vi "DMM_Keysight_34980A_SoftFP.vi"(0 "reference in":refnum<class "DMM_Keysight_34980A.lvclass">, 2 "Floating":bool, 5 "error in (no error)":errorcluster) -> (14 "reference out":refnum<class "DMM_Keysight_34980A.lvclass">, 19 "error out":errorcluster)   [LabVIEW 2022 SP3, in "DMM_Keysight_34980A.lvlib" / "DMM_Keysight_34980A.lvclass"]
uses:
  DMM_Keysight_34980A.lvclass
  Res.ctl
  Mode.ctl
  <vilib>/Analysis/baseanly.llb/Mean (DBL).vi
  Components/ViPER.lvlibp/ViPER.lvclass
  <vilib>/Utility/Data Type/NI_Data Type.lvlib
  C:/Projects/Medulla/ViPER/Examples/Flux_Capacitor_Tester/Components/ViPER.lvlibp/ViPER.lvclass
  <vilib>/Analysis/NI_AALBase.lvlib
panel:
  out "result":dbl
  in  "BW or low F":string(combo) caption="Combo Box"
  in  "Aperature":string(combo) caption="Combo Box"
  in  "Range":string(combo) caption="Combo Box"
  in  "Mode":string(combo) caption="Combo Box"
  in  "Resolution":string(combo) caption="Combo Box"
  in  "Timeout (s)":dbl=10.0 caption="Numeric" min=10.0 max=360.0 step=1.0
  in  "dt (s)":dbl=0.001 caption="Numeric" min=0.001 max=1.0 step=0.001 format="%_1g"
  in  "Samples":u32=1 caption="Numeric" min=1 max=1500 step=1
  in  "Measure":bool
  out "XY Graph":cluster{"Time":dbl[], "Measurement":dbl[]}(graph)
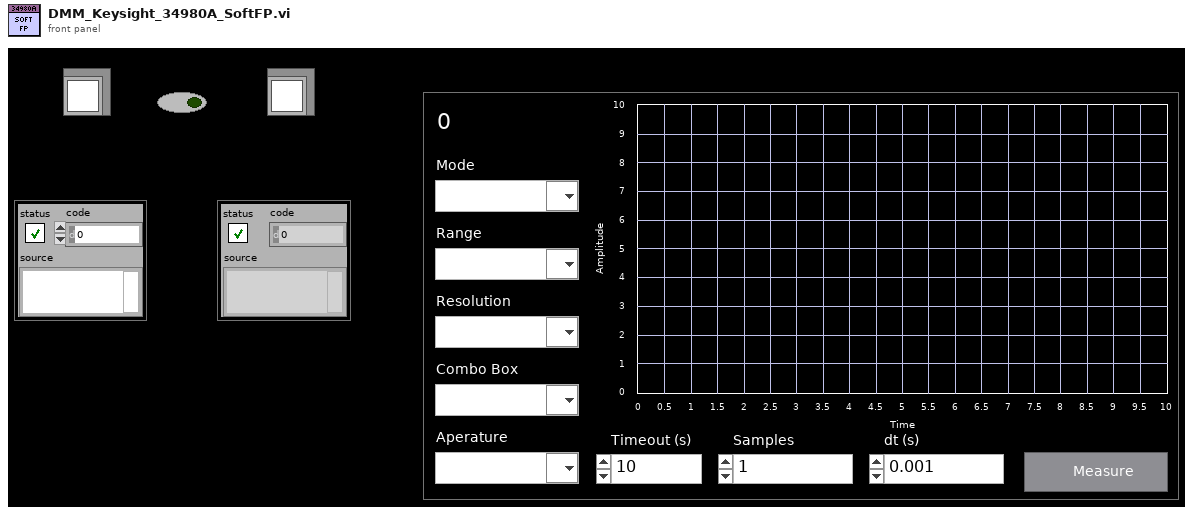
[diagram p1: front panel]
types:
  T1 = enum32{"Invalid", "Standard", "Closed", "Hidden", "Minimized", "Maximized"}
  T2 = enum16{"100 mV", "1 V", "10 V", "100 V", "300 V", "Auto", "Minimum", "Maximum"}
  T3 = enum16{"4 1/2", "5 1/2", "6 1/2", "Least", "Highest", "Default"}
  T4 = enum16{"3 Hz", "20 Hz", "200 Hz", "Minimum", "Maximum"}
  T5 = enum16{"100 mV", "1 V", "10 V", "100 V", "300 V", "Auto", "Minimum", "Maximum", "Default"}
  T6 = enum16{"100 Ohm", "1 kOhm", "10 kOhm", "100 kOhm", "1 MOhm", "10 MOhm", "100 MOhm", "Auto", "Minimum", "Maximum"}
  T7 = enum16{"10 ms", "100 ms", "1 sec", "Minimum", "Maximum"}
  T8 = enum16{"10 mA", "100 mA", "1 A", "Auto", "Minimum", "Maximum"}
  T9 = enum16{"3 Hz", "20 Hz", "200 Hz", "Minimum", "Maximum", "Default"}
  T10 = typedef "DMM_Keysight_34980A.lvlib/DMM_Keysight_34980A.lvclass/Mode.ctl" = enum16{"DCV", "ACV", "2W Ohms", "4W Ohms", "Frequency", "DCA", "ACA"}
  T11 = typedef "DMM_Keysight_34980A.lvlib/DMM_Keysight_34980A.lvclass/Res.ctl" = enum16{"4 1/2", "5 1/2", "6 1/2", "Least", "Highest", "Default"}
  T12 = typedef "DMM_Keysight_34980A.lvlib/DMM_Keysight_34980A.lvclass/ObjectAttributes.ctl" = cluster{"Config":T13, "VISA ref":refnum<visa-resource-name>, "Meas":dbl, "Range DCV":enum16{"100 mV", "1 V", "10 V", "100 V", "300 V", "Auto", "Minimum", "Maximum"}, "Range ACV":enum16{"100 mV", "1 V", "10 V", "100 V", "300 V", "Auto", "Minimum", "Maximum", "Default"}, "Range Ohms":enum16{"100 Ohm", "1 kOhm", "10 kOhm", "100 kOhm", "1 MOhm", "10 MOhm", "100 MOhm", "Auto", "Minimum", "Maximum"}, "Range VFreq":enum16{"100 mV", "1 V", "10 V", "100 V", "300 V", "Auto", "Minimum", "Maximum"}, " Range ACA":enum16{"10 mA", "100 mA", "1 A", "Auto", "Minimum", "Maximum"}, " Range DCA":enum16{"10 mA", "100 mA", "1 A", "Auto", "Minimum", "Maximum"}, "Mode":T10, "Resolution":enum16{"4 1/2", "5 1/2", "6 1/2", "Least", "Highest", "Default"}, "Bandwidth":enum16{"3 Hz", "20 Hz", "200 Hz", "Minimum", "Maximum"}, "Low Frequency":enum16{"3 Hz", "20 Hz", "200 Hz", "Minimum", "Maximum"}, "Aperture":enum16{"10 ms", "100 ms", "1 sec", "Minimum", "Maximum"}, "Measurement":dbl[], "Time":dbl[], "Samples":u32, "dt":dbl, "Timeout":dbl}
  T13 = typedef "DMM_Keysight_34980A.lvlib/DMM_Keysight_34980A.lvclass/Config.ctl" = cluster{"VISA":refnum<visa-resource-name>}
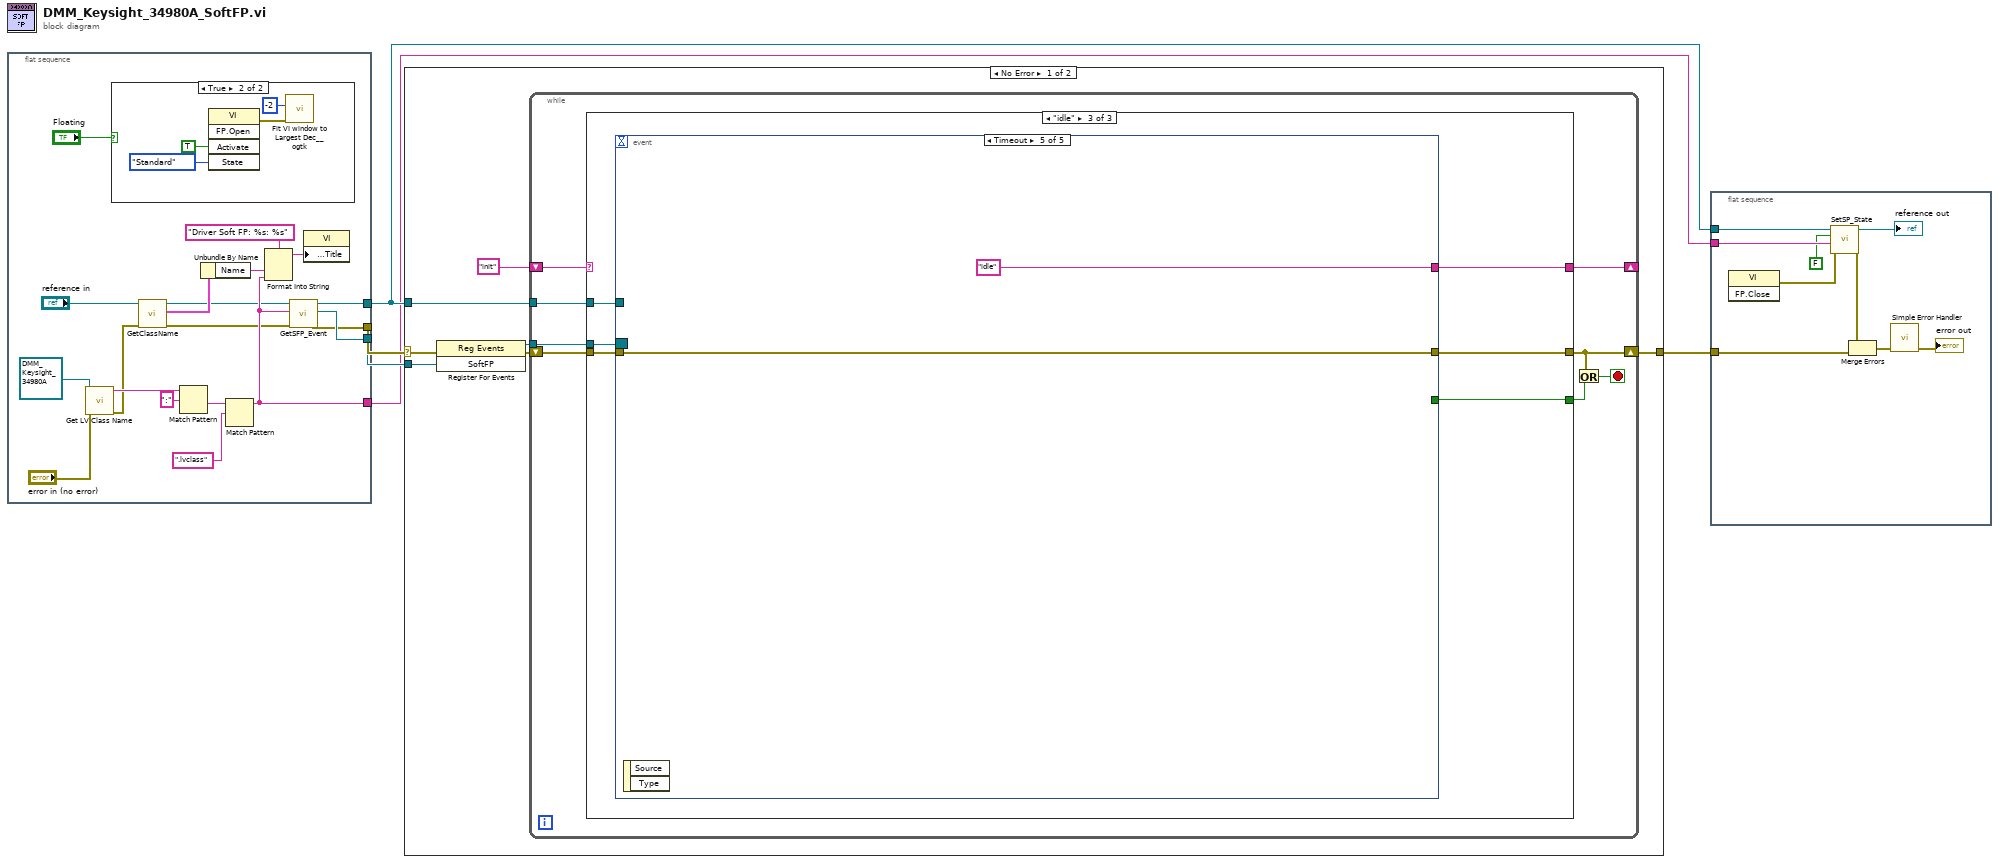
[diagram p0: block diagram]
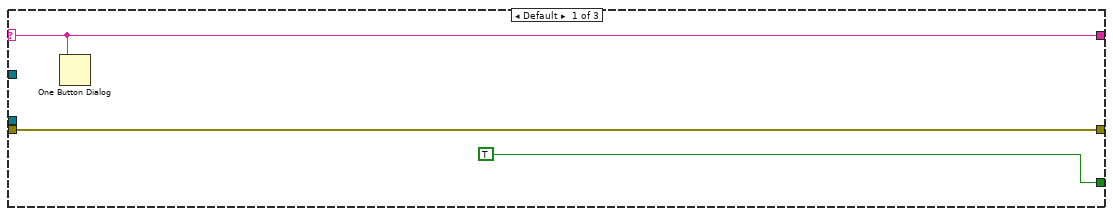
[diagram p3: hidden frame]
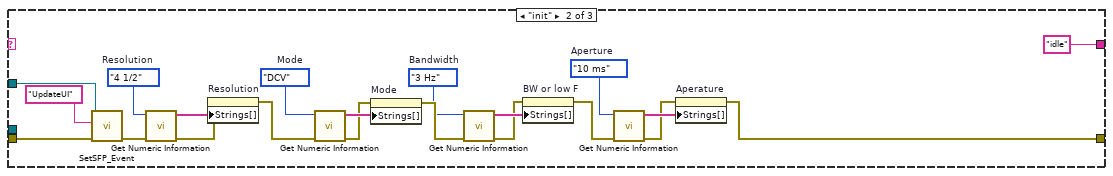
[diagram p4: hidden frame]
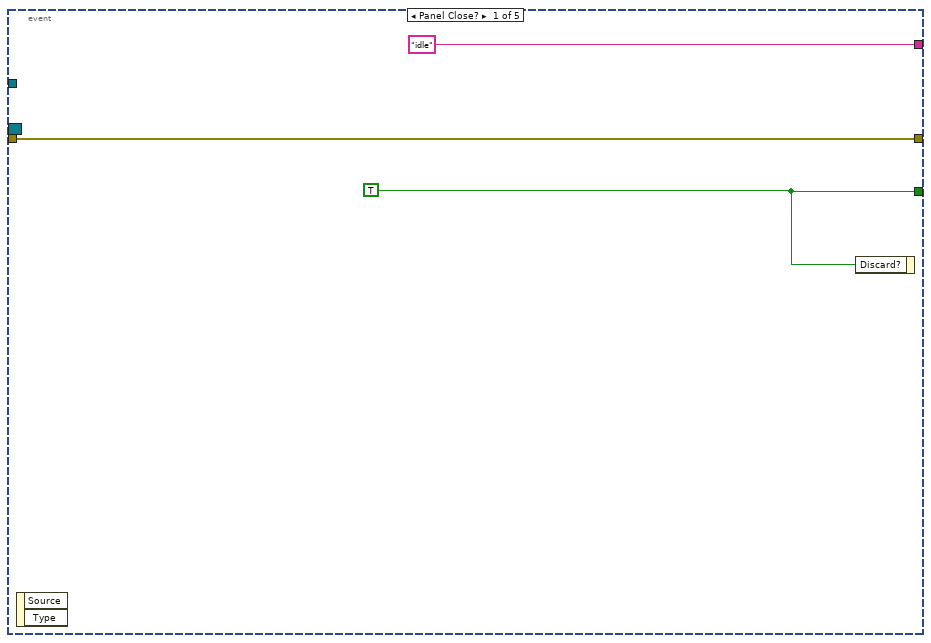
[diagram p5: hidden frame]
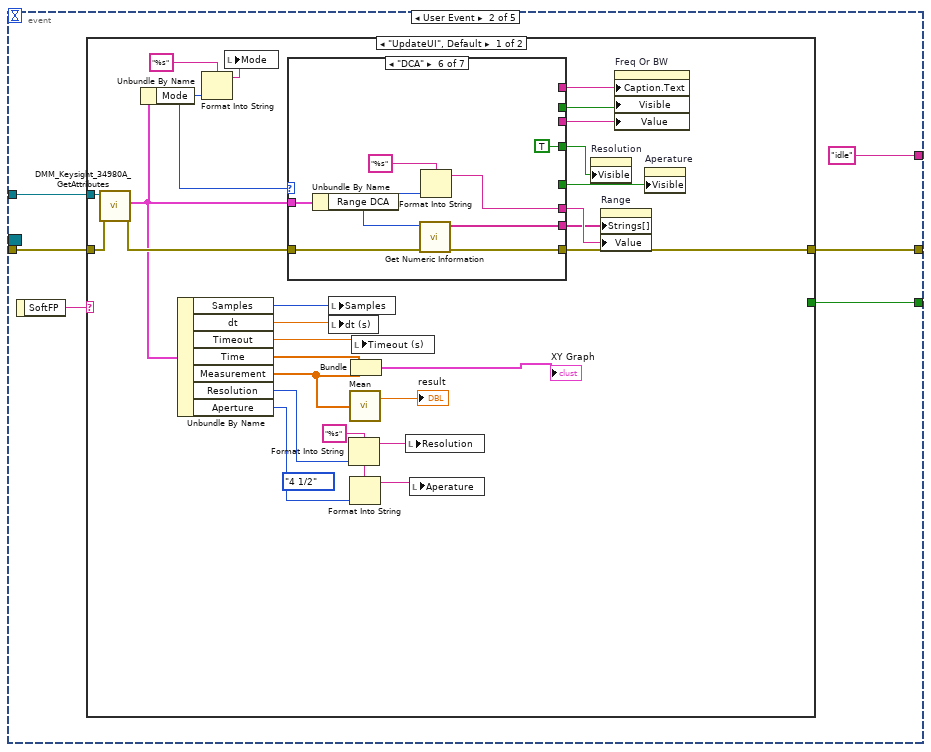
[diagram p6: hidden frame]
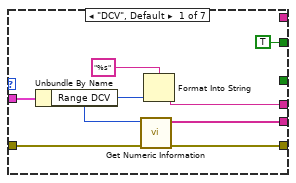
[diagram p7: hidden frame]
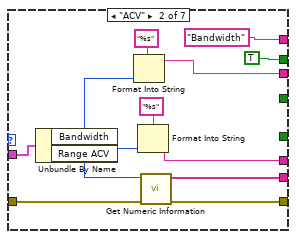
[diagram p8: hidden frame]
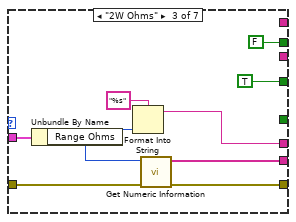
[diagram p9: hidden frame]
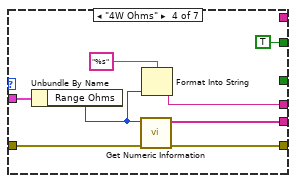
[diagram p10: hidden frame]
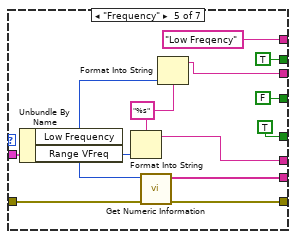
[diagram p11: hidden frame]
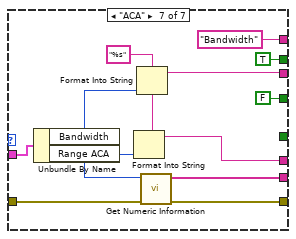
[diagram p12: hidden frame]
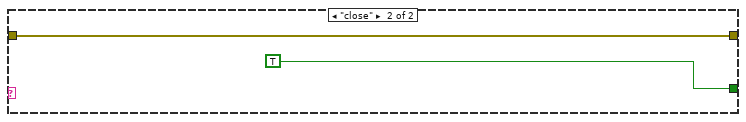
[diagram p13: hidden frame]
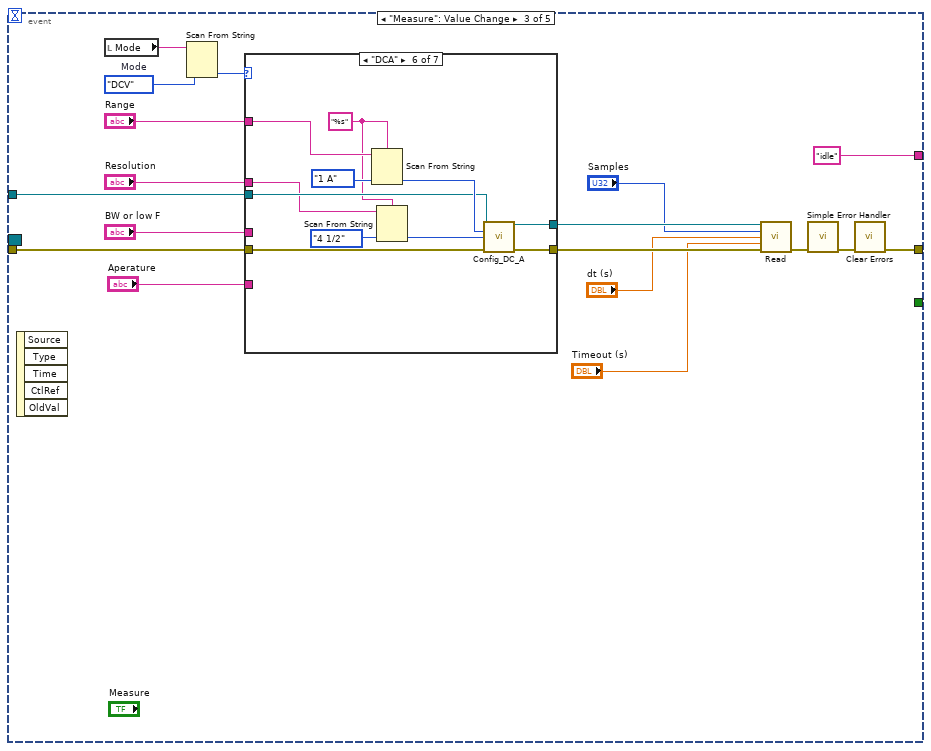
[diagram p14: hidden frame]
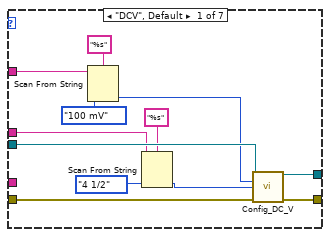
[diagram p15: hidden frame]
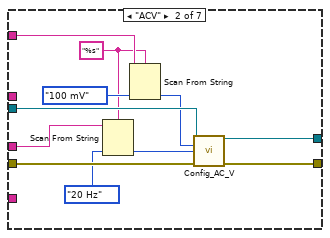
[diagram p16: hidden frame]
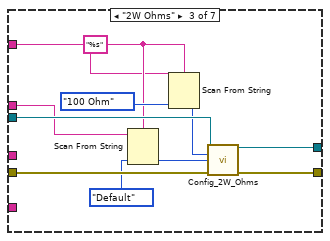
[diagram p17: hidden frame]
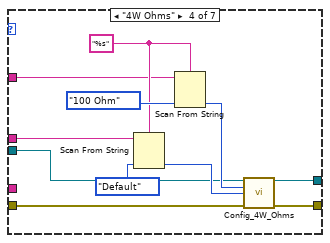
[diagram p18: hidden frame]
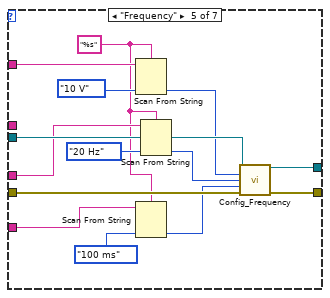
[diagram p19: hidden frame]
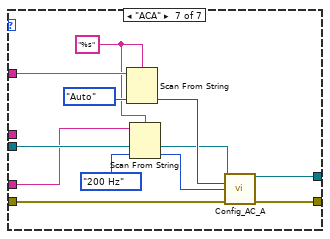
[diagram p20: hidden frame]
diagram:
  n1 = flat-sequence {
    tunnel: [w21] -> w5
    tunnel: [w20] -> w2
    tunnel: [w24] -> w3
    tunnel: [w12] -> w1
    frame #0 {
      n2 = call <vilib>:"Get LV Class Name.vi"("error in (no error)"="error in (no error)", "object"=refnum<class "DMM_Keysight_34980A.lvclass"> refnum ("reference")) -> ("error out"=w11:errorcluster, "class name"=w17:string)  [unwired: 8 in]
      n3 = case shown="True" "Floating" {
        frame False {
        }
        frame True {
          n4 = invoke class="VI" method="FP.Open"("Activate"=TRUE ("Activate?"), "State"=T1."Standard") -> (error out=w25:errorcluster)  [unwired: 3 in, 4 out]
          n5 = call <userlib>:"Fit VI window to Largest Dec__ogtk.vi"("error in (no error)"=w25, "border spacing (2 px)"=-2) -> ()  [unwired: 4 in, 2 out]
        }
      }
      n6 = call "GetClassName.vi"("error in (no error)"=w11, "reference in"="reference in") -> ("error out"=w10:errorcluster, "Details"=w9:cluster{"Name":string, "Class":string}, "reference out"=w7:refnum<class "DMM_Keysight_34980A.lvclass">)  [unwired: 7 in]
      n7 = Match Pattern(string=w17, regular expression=":") -> (after substring=w15:string)  [unwired: 1 in, 3 out]
      n8 = Unbundle By Name(w9) -> ("Name"=w19:string)
      n9 = Match Pattern(string=w15, regular expression=".lvclass") -> (before substring=w12:string)  [unwired: 1 in, 3 out]
      n10 = Format Into String(format string="Driver Soft FP: %s: %s", w19, w12) -> (resulting string=w23:string)  [unwired: 2 in, 1 out]
      n11 = call-dynamic "GetSFP_Event.vi"("error in (no error)"=w10, "Ancestor"=w12, "reference in"=w7) -> ("error out"=w21:errorcluster, "SoftFP"=w24:refnum<user-event>, "reference out"=w20:refnum<class "DMM_Keysight_34980A.lvclass">)  [unwired: 6 in]
      n12 = property class="VI"("Front Panel.Title"=w23) -> ()  [unwired: 2 in, 2 out]
    }
  }
  n13 = case shown="No Error" w5 {
    selector: w5 -> [w33 w301]
    tunnel: [w29 w301] -> w4
    tunnel: w2 -> [w30 _]
    tunnel: w3 -> [w35 _]
    frame No Error {
      n14 = register-events(error in=w33, w35) -> (reference out=w34:refnum<event-registration>, error out=w32:errorcluster)  [unwired: 1 in]
      n15 = while {
        shift-right: [w40] -> w29
        shift-left: w32 -> [w43]
        tunnel: w34 -> [w42]
        tunnel: w30 -> [w41]
        shift-right: [w36] -> _
        shift-left: "init" -> [w37]
        stop <- w39 stop-if-true
        n16 = case shown="\"idle\"" w37 {
          selector: w37 -> [w44 _ _]
          tunnel: w43 -> [w45 w66 w73]
          tunnel: w42 -> [_ _ w72]
          tunnel: w41 -> [_ w65 w71]
          tunnel: [w45 w47 w70] -> w40
          tunnel: [TRUE ("Discard?") _ w69] -> w38
          tunnel: [w44 "idle" w68] -> w36
          frame Default {
            n17 = One Button Dialog(message=w44) -> ()  [unwired: 1 in, 1 out]
          }
          frame "init" {
            w50 = T7."10 ms"  # Aperture
            w54 = T4."3 Hz"  # Bandwidth
            w58 = Mode."DCV"  # Mode
            w62 = Res."4 1/2"  # Resolution
            n18 = call-dynamic "SetSFP_Event.vi"("error in (no error)"=w66, "msg"="UpdateUI", "reference in"=w65) -> ("error out"=w63:errorcluster)  [unwired: 7 in, 1 out]
            n19 = call <vilib>:"Get Numeric Information.vi"("error in (no error)"=w63, "variant"=w62) -> ("error out"=w60:errorcluster, "enum names"=w61:string[])  [unwired: 6 in, 2 out]
            n20 = property on="Resolution" class="CmbBox"(error in=w60, "Strings[]"=w61) -> (error out=w59:errorcluster)  [unwired: 1 in, 1 out]
            n21 = call <vilib>:"Get Numeric Information.vi"("error in (no error)"=w59, "variant"=w58) -> ("error out"=w56:errorcluster, "enum names"=w57:string[])  [unwired: 6 in, 2 out]
            n22 = property on="Mode" class="CmbBox"(error in=w56, "Strings[]"=w57) -> (error out=w55:errorcluster)  [unwired: 1 in, 1 out]
            n23 = call <vilib>:"Get Numeric Information.vi"("error in (no error)"=w55, "variant"=w54) -> ("error out"=w52:errorcluster, "enum names"=w53:string[])  [unwired: 6 in, 2 out]
            n24 = property on="BW or low F" class="CmbBox"(error in=w52, "Strings[]"=w53) -> (error out=w51:errorcluster)  [unwired: 1 in, 1 out]
            n25 = call <vilib>:"Get Numeric Information.vi"("error in (no error)"=w51, "variant"=w50) -> ("error out"=w48:errorcluster, "enum names"=w49:string[])  [unwired: 6 in, 2 out]
            n26 = property on="Aperature" class="CmbBox"(error in=w48, "Strings[]"=w49) -> (error out=w47:errorcluster)  [unwired: 1 in, 1 out]
          }
          frame "idle" {
            n27 = event shown="[4] Timeout" {
              selector: w72 -> [_ _ _ _ _]
              dyn-events: _ -> [_ _ _ _ _]
              timeout: _ -> [_ _ _ _ _]
              tunnel: w73 -> [w76 w82 w199 w289 w300]
              tunnel: [w76 w80 w184 w291 w300] -> w70
              tunnel: [w75 w79 _ _ _] -> w69
              tunnel: w71 -> [_ w77 w198 w288 _]
              tunnel: ["idle" "idle" "idle" "idle" "idle"] -> w68
              event Panel Close? {
                w75 = TRUE ("Discard?")
                n28 = event-data() -> ()  [unwired: 1 in, 2 out]
                n29 = event-data("Discard?"=w75) -> ()  [unwired: 1 in, 1 out]
              }
              event User Event {
                n30 = event-data() -> ("SoftFP"=w81:string)  [unwired: 1 in]
                n31 = case shown="\"UpdateUI\", Default" w81 {
                  tunnel: w82 -> [w109 w181]
                  tunnel: [w107 w181] -> w80
                  tunnel: [_ TRUE ("Discard?")] -> w79
                  tunnel: w77 -> [w108 _]
                  frame "UpdateUI", Default {
                    (unwired) T3."4 1/2" ("Resolution")
                    w86 = "%s" ("format string")
                    n32 = call "DMM_Keysight_34980A_GetAttributes.vi"("error in (no error)"=w109, "reference in"=w108) -> ("error out"=w97:errorcluster, "Data"=w96:T12)  [unwired: 6 in, 2 out]
                    n33 = Unbundle By Name(w96) -> ("Mode"=w104:T10)
                    n34 = Unbundle By Name(w96) -> ("Samples"=w95:u32, "dt"=w94:dbl, "Timeout"=w93:dbl, "Time"=w92:dbl[], "Measurement"=w91:dbl[], "Resolution"=w88:T3, "Aperture"=w85:T7)
                    n35 = Format Into String(format string="%s", w104) -> (resulting string=w103:string)  [unwired: 2 in, 1 out]
                    n36 = local write "Mode"(w103) -> ()
                    n37 = case shown="\"DCA\"" w104 {
                      tunnel: w96 -> [w115 w127 w136 w144 w157 w165 w177]
                      tunnel: w97 -> [w117 w129 w138 w146 w159 w167 w179]
                      tunnel: [w116 w128 w137 w145 w158 w166 w178] -> w107
                      tunnel: [w112 w124 w133 w141 w155 w163 w175] -> w105
                      tunnel: [w111 w123 w132 w140 w154 w160 w174] -> w106
                      tunnel: [_ "Bandwidth" _ _ "Low Freqency" _ "Bandwidth"] -> w101
                      tunnel: [_ TRUE FALSE _ TRUE _ TRUE] -> w100
                      tunnel: [TRUE _ TRUE TRUE FALSE TRUE FALSE] -> w99
                      tunnel: [_ _ _ _ TRUE _ _] -> w98
                      tunnel: [_ w118 _ _ w147 _ w171] -> w89
                      frame "DCV", Default {
                        n38 = Unbundle By Name(w115) -> ("Range DCV"=w113:T2)
                        n39 = call <vilib>:"Get Numeric Information.vi"("error in (no error)"=w117, "variant"=w113) -> ("error out"=w116:errorcluster, "enum names"=w112:string[])  [unwired: 6 in, 2 out]
                        n40 = Format Into String(format string="%s", w113) -> (resulting string=w111:string)  [unwired: 2 in, 1 out]
                      }
                      frame "ACV" {
                        n41 = Unbundle By Name(w127) -> ("Bandwidth"=w119:T4, "Range ACV"=w125:T5)
                        n42 = Format Into String(format string="%s", w119) -> (resulting string=w118:string)  [unwired: 2 in, 1 out]
                        n43 = Format Into String(format string="%s", w125) -> (resulting string=w123:string)  [unwired: 2 in, 1 out]
                        n44 = call <vilib>:"Get Numeric Information.vi"("error in (no error)"=w129, "variant"=w125) -> ("error out"=w128:errorcluster, "enum names"=w124:string[])  [unwired: 6 in, 2 out]
                      }
                      frame "2W Ohms" {
                        n45 = Unbundle By Name(w136) -> ("Range Ohms"=w134:T6)
                        n46 = Format Into String(format string="%s", w134) -> (resulting string=w132:string)  [unwired: 2 in, 1 out]
                        n47 = call <vilib>:"Get Numeric Information.vi"("error in (no error)"=w138, "variant"=w134) -> ("error out"=w137:errorcluster, "enum names"=w133:string[])  [unwired: 6 in, 2 out]
                      }
                      frame "4W Ohms" {
                        n48 = Unbundle By Name(w144) -> ("Range Ohms"=w142:T6)
                        n49 = call <vilib>:"Get Numeric Information.vi"("error in (no error)"=w146, "variant"=w142) -> ("error out"=w145:errorcluster, "enum names"=w141:string[])  [unwired: 6 in, 2 out]
                        n50 = Format Into String(format string="%s", w142) -> (resulting string=w140:string)  [unwired: 2 in, 1 out]
                      }
                      frame "Frequency" {
                        w149 = "%s" ("format string")
                        n51 = Unbundle By Name(w157) -> ("Low Frequency"=w148:T4, "Range VFreq"=w156:T2)
                        n52 = Format Into String(format string=w149, w156) -> (resulting string=w154:string)  [unwired: 2 in, 1 out]
                        n53 = call <vilib>:"Get Numeric Information.vi"("error in (no error)"=w159, "variant"=w156) -> ("error out"=w158:errorcluster, "enum names"=w155:string[])  [unwired: 6 in, 2 out]
                        n54 = Format Into String(format string=w149, w148) -> (resulting string=w147:string)  [unwired: 2 in, 1 out]
                      }
                      frame "DCA" {
                        n55 = Unbundle By Name(w165) -> ("Range DCA"=w164:T8)
                        n56 = call <vilib>:"Get Numeric Information.vi"("error in (no error)"=w167, "variant"=w164) -> ("error out"=w166:errorcluster, "enum names"=w163:string[])  [unwired: 6 in, 2 out]
                        n57 = Format Into String(format string="%s", w164) -> (resulting string=w160:string)  [unwired: 2 in, 1 out]
                      }
                      frame "ACA" {
                        w168 = "%s" ("format string")
                        n58 = Unbundle By Name(w177) -> ("Bandwidth"=w172:T4, "Range ACA"=w176:T8)
                        n59 = Format Into String(format string=w168, w176) -> (resulting string=w174:string)  [unwired: 2 in, 1 out]
                        n60 = Format Into String(format string=w168, w172) -> (resulting string=w171:string)  [unwired: 2 in, 1 out]
                        n61 = call <vilib>:"Get Numeric Information.vi"("error in (no error)"=w179, "variant"=w176) -> ("error out"=w178:errorcluster, "enum names"=w175:string[])  [unwired: 6 in, 2 out]
                      }
                    }
                    n62 = local write "Samples"(w95) -> ()
                    n63 = local write "dt (s)"(w94) -> ()
                    n64 = Format Into String(format string=w86, w88) -> (resulting string=w87:string)  [unwired: 2 in, 1 out]
                    n65 = call-poly <vilib>:"Mean.vi"("X"=w91) -> ("mean"=→"result":dbl)  [unwired: 1 out]
                    n66 = Format Into String(format string=w86, w85) -> (resulting string=w84:string)  [unwired: 2 in, 1 out]
                    n67 = Bundle("Time"=w92, "Measurement"=w91) -> (→"XY Graph":cluster{"Time":dbl[], "Measurement":dbl[]})  [unwired: 1 in]
                    n68 = local write "Timeout (s)"(w93) -> ()
                    n69 = local write "Resolution"(w87) -> ()
                    n70 = local write "Aperature"(w84) -> ()
                    n71 = property on="Resolution" class="CmbBox"("Visible"=w99) -> ()  [unwired: 2 in, 2 out]
                    n72 = property on="Range" class="CmbBox"("Strings[]"=w105, "Value"=w106) -> ()  [unwired: 2 in, 2 out]
                    n73 = property on="Freq Or BW" class="CmbBox"("Caption.Text"=w101, "Visible"=w100, "Value"=w89) -> ()  [unwired: 2 in, 2 out]
                    n74 = property on="Aperature" class="CmbBox"("Visible"=w98) -> ()  [unwired: 2 in, 2 out]
                  }
                  frame "close" {
                  }
                }
              }
              event "Measure": Value Change {
                w191 = Mode."DCV"  # Mode
                n75 = event-data() -> ()  [unwired: 1 in, 5 out]
                n76 = local read "Mode"() -> (w189:string)
                n77 = Scan From String(input string=w189, default 1=w191) -> (output 1=w190:T10)  [unwired: 3 in, 3 out]
                n78 = case shown="\"DCA\"" w190 {
                  tunnel: w199 -> [w210 w222 w233 w244 w258 w269 w280]
                  tunnel: w198 -> [w209 w221 w232 w234 w257 w265 w276]
                  tunnel: "Resolution" -> [w203 _ w223 w238 _ w261 _]
                  tunnel: [w208 w218 w229 w243 w254 w268 w279] -> w195
                  tunnel: [w207 w217 w228 w242 w253 w264 w275] -> w194
                  tunnel: "Range" -> [w205 w216 w224 w237 w252 w263 w274]
                  tunnel: "BW or low F" -> [_ w215 _ _ w251 _ w272]
                  tunnel: "Aperature" -> [_ _ _ _ w247 _ _]
                  frame "DCV", Default {
                    n79 = Scan From String(format string="%s", input string=w205, default 1=T2."100 mV" ("Range (5:Auto)")) -> (output 1=w204:T2)  [unwired: 2 in, 3 out]
                    n80 = Scan From String(format string="%s", input string=w203, default 1=T3."4 1/2" ("Resolution (5:Default)")) -> (output 1=w200:T3)  [unwired: 2 in, 3 out]
                    n81 = call-dynamic "Config_DC_V.vi"("reference in"=w209, "Range (5:Auto)"=w204, "Resolution (5:Default)"=w200, "error in (no error)"=w210) -> ("reference in"=w207:refnum<class "DMM_Keysight_34980A.lvclass">, "error out"=w208:errorcluster)  [unwired: 10 in]
                  }
                  frame "ACV" {
                    w212 = "%s" ("format string")
                    n82 = Scan From String(format string=w212, input string=w215, default 1=T4."20 Hz" ("Bandwidth (1:20 Hz)")) -> (output 1=w213:T4)  [unwired: 2 in, 3 out]
                    n83 = Scan From String(format string=w212, input string=w216, default 1=T5."100 mV" ("Range (5:Auto)")) -> (output 1=w219:T5)  [unwired: 2 in, 3 out]
                    n84 = call-dynamic "Config_AC_V.vi"("reference in"=w221, "Range (5:Auto)"=w219, "Bandwidth (1:20 Hz)"=w213, "error in (no error)"=w222) -> ("reference in"=w217:refnum<class "DMM_Keysight_34980A.lvclass">, "error out"=w218:errorcluster)  [unwired: 10 in]
                  }
                  frame "2W Ohms" {
                    w227 = "%s" ("format string")
                    n85 = Scan From String(format string=w227, input string=w223, default 1=T3."Default" ("Resolution (5:Default)")) -> (output 1=w225:T3)  [unwired: 2 in, 3 out]
                    n86 = Scan From String(format string=w227, input string=w224, default 1=T6."100 Ohm" ("Range (7:Auto)")) -> (output 1=w230:T6)  [unwired: 2 in, 3 out]
                    n87 = call-dynamic "Config_2W_Ohms.vi"("reference in"=w232, "Range (7:Auto)"=w230, "Resolution (5:Default)"=w225, "error in (no error)"=w233) -> ("reference in"=w228:refnum<class "DMM_Keysight_34980A.lvclass">, "error out"=w229:errorcluster)  [unwired: 10 in]
                  }
                  frame "4W Ohms" {
                    w240 = "%s" ("format string")
                    n88 = Scan From String(format string=w240, input string=w238, default 1=T3."Default" ("Resolution (5:Default)")) -> (output 1=w236:T3)  [unwired: 2 in, 3 out]
                    n89 = Scan From String(format string=w240, input string=w237, default 1=T6."100 Ohm" ("Range (7:Auto)")) -> (output 1=w235:T6)  [unwired: 2 in, 3 out]
                    n90 = call-dynamic "Config_4W_Ohms.vi"("reference in"=w234, "Range (7:Auto)"=w235, "Resolution (5:Default)"=w236, "error in (no error)"=w244) -> ("reference in"=w242:refnum<class "DMM_Keysight_34980A.lvclass">, "error out"=w243:errorcluster)  [unwired: 10 in]
                  }
                  frame "Frequency" {
                    w248 = "%s" ("format string")
                    n91 = Scan From String(format string=w248, input string=w252, default 1=T2."10 V" ("Voltage Range (5:Auto)")) -> (output 1=w255:T2)  [unwired: 2 in, 3 out]
                    n92 = Scan From String(format string=w248, input string=w247, default 1=T7."100 ms" ("Aperture (1:100 ms)")) -> (output 1=w245:T7)  [unwired: 2 in, 3 out]
                    n93 = Scan From String(format string=w248, input string=w251, default 1=T4."20 Hz" ("Low Frequency (1:20 Hz)")) -> (output 1=w249:T4)  [unwired: 2 in, 3 out]
                    n94 = call-dynamic "Config_Frequency.vi"("reference in"=w257, "Voltage Range (5:Auto)"=w255, "Low Frequency (1:20 Hz)"=w249, "Aperture (1:100 ms)"=w245, "error in (no error)"=w258) -> ("reference in"=w253:refnum<class "DMM_Keysight_34980A.lvclass">, "error out"=w254:errorcluster)  [unwired: 9 in]
                  }
                  frame "DCA" {
                    w260 = "%s" ("format string")
                    n95 = Scan From String(format string=w260, input string=w263, default 1=T8."1 A" ("Range (3:Auto)")) -> (output 1=w266:T8)  [unwired: 2 in, 3 out]
                    n96 = Scan From String(format string=w260, input string=w261, default 1=T3."4 1/2" ("Resolution (5:Default)")) -> (output 1=w259:T3)  [unwired: 2 in, 3 out]
                    n97 = call-dynamic "Config_DC_A.vi"("reference in"=w265, "Range (3:Auto)"=w266, "Resolution (5:Default)"=w259, "error in (no error)"=w269) -> ("reference in"=w264:refnum<class "DMM_Keysight_34980A.lvclass">, "error out"=w268:errorcluster)  [unwired: 10 in]
                  }
                  frame "ACA" {
                    w273 = "%s" ("format string")
                    n98 = Scan From String(format string=w273, input string=w274, default 1=T8."Auto" ("Range (3:Auto)")) -> (output 1=w277:T8)  [unwired: 2 in, 3 out]
                    n99 = Scan From String(format string=w273, input string=w272, default 1=T9."200 Hz" ("Bandwidth (5:Default)")) -> (output 1=w270:T9)  [unwired: 2 in, 3 out]
                    n100 = call-dynamic "Config_AC_A.vi"("reference in"=w276, "Range (3:Auto)"=w277, "Bandwidth (5:Default)"=w270, "error in (no error)"=w280) -> ("reference in"=w275:refnum<class "DMM_Keysight_34980A.lvclass">, "error out"=w279:errorcluster)  [unwired: 10 in]
                  }
                }
                n101 = call-dynamic "Read.vi"("reference in"=w194, "Samples"="Samples", "dt"="dt (s)", "Timeout (10 s)"="Timeout (s)", "error in (no error)"=w195) -> ("error out"=w186:errorcluster)  [unwired: 7 in, 3 out]
                n102 = call <vilib>:"Simple Error Handler.vi"("error in (no error)"=w186) -> ("error out"=w185:errorcluster)  [unwired: 4 in, 4 out]
                n103 = call <vilib>:"Clear Errors.vi"("error in (no error)"=w185) -> ("error out"=w184:errorcluster)  [unwired: 5 in, 1 out]
              }
              event "Mode": Value Change {
                w283 = Mode."DCV"  # Mode
                n104 = event-data() -> ()  [unwired: 1 in, 5 out]
                n105 = call "DMM_Keysight_34980A_GetAttributes.vi"("error in (no error)"=w289, "reference in"=w288) -> ("error out"=w290:errorcluster, "DataRef"=w287:refnum<data-value>, "reference out"=w285:refnum<class "DMM_Keysight_34980A.lvclass">)  [unwired: 6 in, 1 out]
                n106 = Scan From String(input string="Mode", default 1=w283) -> (output 1=w281:T10)  [unwired: 3 in, 3 out]
                n107 = in-place {
                  in-place-border: w281 -> [w296]
                  n108 = in-place-dvr #1(w287) -> (w298:T12)  [unwired: 1 out]
                  n109 = Bundle By Name(cluster=w298, "Mode"=w296) -> (w297:T12)
                  n110 = in-place-dvr #1(w297) -> (w286:errorcluster)  [unwired: 1 out]
                }
                n111 = flat-sequence {
                  tunnel: [w295] -> w291
                  tunnel: w290 -> [w294]
                  tunnel: w286 -> [_]
                  tunnel: w285 -> [w293]
                  frame #0 {
                    n112 = call-dynamic "SetSFP_Event.vi"("error in (no error)"=w294, "msg"="UpdateUI", "reference in"=w293) -> ("error out"=w295:errorcluster)  [unwired: 7 in, 1 out]
                  }
                }
              }
              event Timeout {
                n113 = event-data() -> ()  [unwired: 1 in, 2 out]
              }
            }
          }
        }
        n114 = Or(x=w40, y=w38) -> (x .or. y?=w39:bool)
      }
    }
    frame Error {
    }
  }
  n115 = flat-sequence {
    tunnel: w4 -> [w308]
    tunnel: w2 -> [w303]
    tunnel: w1 -> [w305]
    frame #0 {
      n116 = invoke class="VI" method="FP.Close"() -> (error out=w307:errorcluster)  [unwired: 3 in, 2 out]
      n117 = call "SetSP_State.vi"("error in (no error)"=w307, "Ancestor"=w305, "SP Open"=FALSE, "reference in"=w303) -> ("error out"=w306:errorcluster, "reference out"=→"reference out":refnum<class "DMM_Keysight_34980A.lvclass">)  [unwired: 6 in]
      n118 = Merge Errors(w306, w308) -> (w310:errorcluster)
      n119 = call <vilib>:"Simple Error Handler.vi"("error in (no error)"=w310) -> ("error out"=→"error out":errorcluster)  [unwired: 4 in, 4 out]
    }
  }
